vi "Teleop.vi"(10 "Match Info":T1={"Autonomous Elapsed Seconds"=0.0, "TeleOp Elapsed Seconds"=0.0, "Disabled Elapsed Seconds"=0.0, "Visited Autonomous"=FALSE, "Visited TeleOp"=FALSE, "Visited Disabled"=FALSE, "Autonomous Settings"={"Autonomous Style"=enum."Independent", "VI Refnum"=refnum}}, 11 "Call Context":T2) -> ()   [LabVIEW 2017]
doc: "This VI is called for each TeleOp packet received from the DS where the robot is not disabled. It is often used to read from the joysticks and update I/O or to update setpoints for timed control loops. It should complete and return within 20 milliseconds or it may miss DS packets."
uses:
  <vilib>/Rock Robotics/WPI/DriverStation/WPI_DriverStationDerivedRobotMode.ctl
  <vilib>/Rock Robotics/WPI/DriverStation/WPI_DriverStationMatch Info.ctl
  <vilib>/Rock Robotics/WPI/Solenoid/WPI_SolenoidValue.ctl
  <vilib>/Rock Robotics/WPI/ThirdParty/Phoenix-LabVIEW/Motor Controller/Controls/CTRE_Phoenix_MotorControl_ControlMode.ctl
  <vilib>/Rock Robotics/WPI/Utilities/WPI_GetSetVariantRefNum.vi
  <vilib>/Rock Robotics/WPI/Solenoid/WPI_SolenoidSetEnum.vi
  <vilib>/Rock Robotics/Network Tables/NT Write Boolean Array.vi
  <vilib>/Rock Robotics/Network Tables/NT Write Numeric Array.vi
  <vilib>/Rock Robotics/Network Tables/NT Read Boolean.vi
  <vilib>/Rock Robotics/Network Tables/NT Read Number.vi
  Robot Global Data.vi
  <vilib>/addons/control/pid/NI_PID_pid.lvlib
  <vilib>/addons/control/pid/pid.llb/PID (DBL).vi
panel:
  out "Claw Status":bool
  out "AbsArm":dbl
  out "Sample Slider 0":dbl(slide) scale=0.0..5.0
  out "Sample Boolean 1":bool
  out "Sample Boolean 0":bool
  # "TUSKS"
  # "Axis 1"
  # "DRIVE"
  # "Axis 1"
  # "PULSE"
  # "Button 3"
  # "Button 3"
  # "Axis 0"
  # "Axis 0"
  # "Button 2"
  # "Button 1"
  # "Button 2"
  # "Button 1"
  # "Button 0"
  # "Button 0"
  # "CONTROLLER  LAYOUT"
  # "CONTROLLER  LAYOUT"
  # "Joystick 1"
  # "Joystick 0"
  # "Joystick 1"
  # "https://www.xbox.com/en-us/xbox-one/accessories"
  # "Axis 4"
  # "Axis 4"
  # "DRIVE TURN"
  # "Left"
  # "Left"
  # "Axis 5"
  # "Axis 5"
  # "CLAW IN"
  # "Button 4"
  # "ELBOW DOWN"
  # "Button 4"
  # "Axis 2"
  # "ARM DOWN"
  # "Axis 2"
  # "BELT IN"
  # "Right"
  # "Button 5"
  # "ELBOW UP"
  # "Button 5"
  # "CLAW OUT"
  # "Axis 3"
  # "ARM UP"
  # "Axis 3"
  # "BELT OUT"
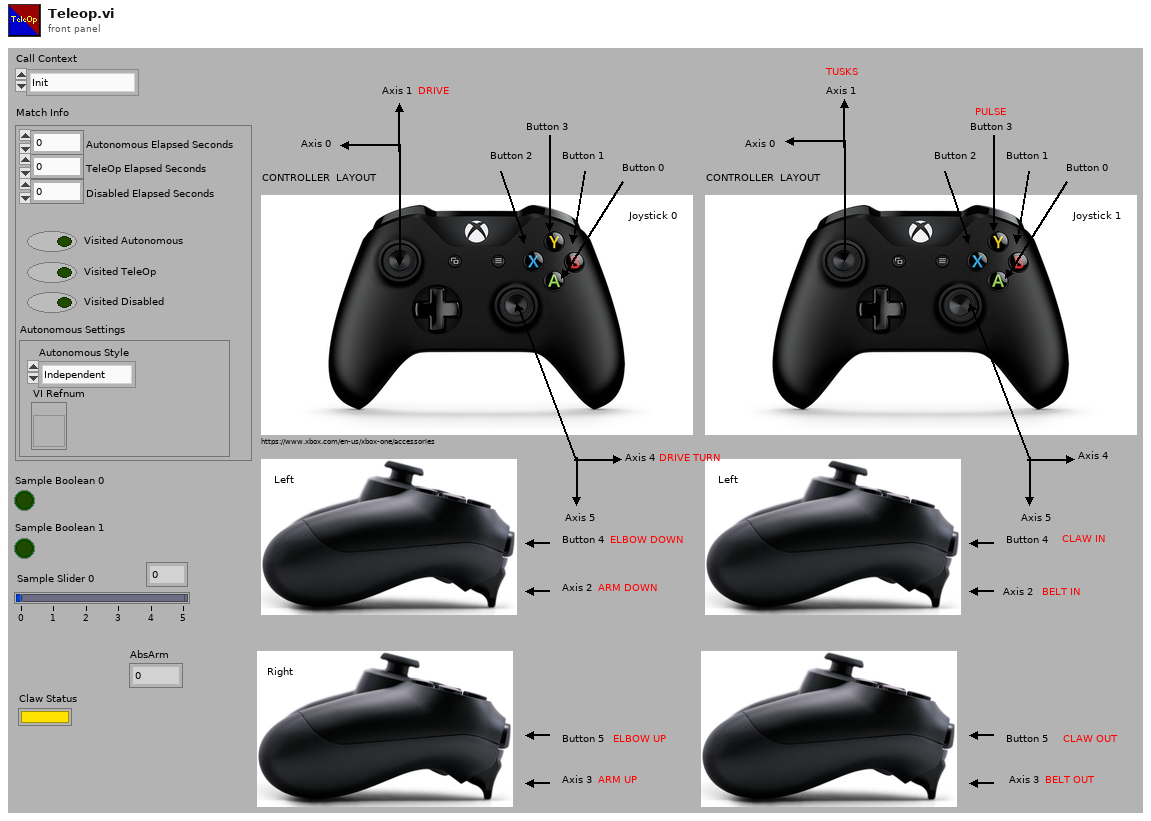
[diagram p1: front panel]
types:
  T1 = typedef "WPI_DriverStationMatch Info.ctl" = cluster{"Autonomous Elapsed Seconds":dbl, "TeleOp Elapsed Seconds":dbl, "Disabled Elapsed Seconds":dbl, "Visited Autonomous":bool, "Visited TeleOp":bool, "Visited Disabled":bool, "Autonomous Settings":cluster{"Autonomous Style":enum16{"Iterative", "Independent"}, "VI Refnum":refnum<vi>}}
  T2 = typedef "WPI_DriverStationDerivedRobotMode.ctl" = enum16{"Init", "Execute", "Stop"}
  T3 = typedef "WPI_JoystickDevRef.ctl" = cluster{"Device":T4}
  T4 = typedef "WPI_JoystickDeviceEnum.ctl" = enum16{"USB 0", "USB 1", "USB 2", "USB 3", "USB 4", "USB 5"}
  T5 = cluster{"Axes[0]":dbl, "Axes[1]":dbl, "Axes[2]":dbl, "Axes[3]":dbl, "Axes[4]":dbl, "Axes[5]":dbl, "Axes[6]":dbl, "Axes[7]":dbl, "Axes[8]":dbl}
  T6 = cluster{"Buttons[0]":bool, "Buttons[1]":bool, "Buttons[2]":bool, "Buttons[3]":bool, "Buttons[4]":bool, "Buttons[5]":bool, "Buttons[6]":bool, "Buttons[7]":bool, "Buttons[8]":bool}
  T7 = typedef "CTRE_Phoenix_MotorControl_ControlMode.ctl" = u16
  T8 = typedef "WPI_MotorControlDeviceRef.ctl" = cluster{"DeviceStatus":errorcluster, "Type":T9, "PWM":cluster{"PWM Channel":T10, "DeadBand":T11}, "CAN":cluster{"Device Number":u8, "SetOutput VI Ref":variant, "GetOutput VI Ref":variant, "Enable VI Ref":variant, "Disable VI Ref":variant, "Data":variant}, "Invert":bool, "DIO PWM":cluster{"PWM \"Enable\" Channel":T10, "DIOChannel":T12, "PWM Rate":dbl}}
  T9 = typedef "WPI_MotorControlType.ctl" = enum16{"PWM", "CAN", "DIO PWM"}
  T10 = typedef "FPGA_DIOPWMChannel.ctl" = enum8{"PWM 0", "PWM 1", "PWM 2", "PWM 3", "PWM 4", "PWM 5", "PWM 6", "PWM 7", "PWM 8", "PWM 9", "PWM MXP 0", "PWM MXP 1", "PWM MXP 2", "PWM MXP 3", "PWM MXP 4", "PWM MXP 5", "PWM MXP 6", "PWM MXP 7", "PWM MXP 8", "PWM MXP 9", "Invalid"}
  T11 = typedef "WPI_PWMDeadband.ctl" = cluster{"Name":string, "maxPositivePwm":i32, "minPositivePwm":i32, "centerPwm":i32, "maxNegativePwm":i32, "minNegativePwm":i32, "angularRange":u16}
  T12 = typedef "FPGA_DIOChannel.ctl" = enum8{"DIO 0", "DIO 1", "DIO 2", "DIO 3", "DIO 4", "DIO 5", "DIO 6", "DIO 7", "DIO 8", "DIO 9", "DIO MXP 0", "DIO MXP 1", "DIO MXP 2", "DIO MXP 3", "DIO MXP 4", "DIO MXP 5", "DIO MXP 6", "DIO MXP 7", "DIO MXP 8", "DIO MXP 9", "DIO MXP 10", "DIO MXP 11", "DIO MXP 12", "DIO MXP 13", "DIO MXP 14", "DIO MXP 15", "SPI Port CS1", "SPI Port CS2", "SPI Port CS3", "SPI Port MISO", "SPI Port MOSI", "Invalid"}
  T13 = typedef "WPI_SolenoidValue.ctl" = enum16{"Off", "On", "Forward", "Reverse"}
  T14 = typedef "WPI_SolenoidDevRef.ctl" = cluster{"DevStatus":errorcluster, "Pneumatics Control Module":u8, "Forward Solenoid Channel":T15, "Reverse Solenoid Channel":T15}
  T15 = typedef "WPI_SolenoidChannel.ctl" = enum8{"Solenoid 0", "Solenoid 1", "Solenoid 2", "Solenoid 3", "Solenoid 4", "Solenoid 5", "Solenoid 6", "Solenoid 7", "Invalid"}
  T16 = enum16{"Arm Down", "Arm Switch", "Arm(Low Scale)", "Arm(Normal Scale)", "Arm(High Scale)", "Hang"}
  T17 = cluster{"proportional gain (Kc)":dbl, "integral time (Ti, min)":dbl, "derivative time (Td, min)":dbl}
  T18 = enum16{"Arm Down", "Arm Switch", "Arm(Low Scale)", "Arm(Normal Scale)", "Arm(High Scale)"}
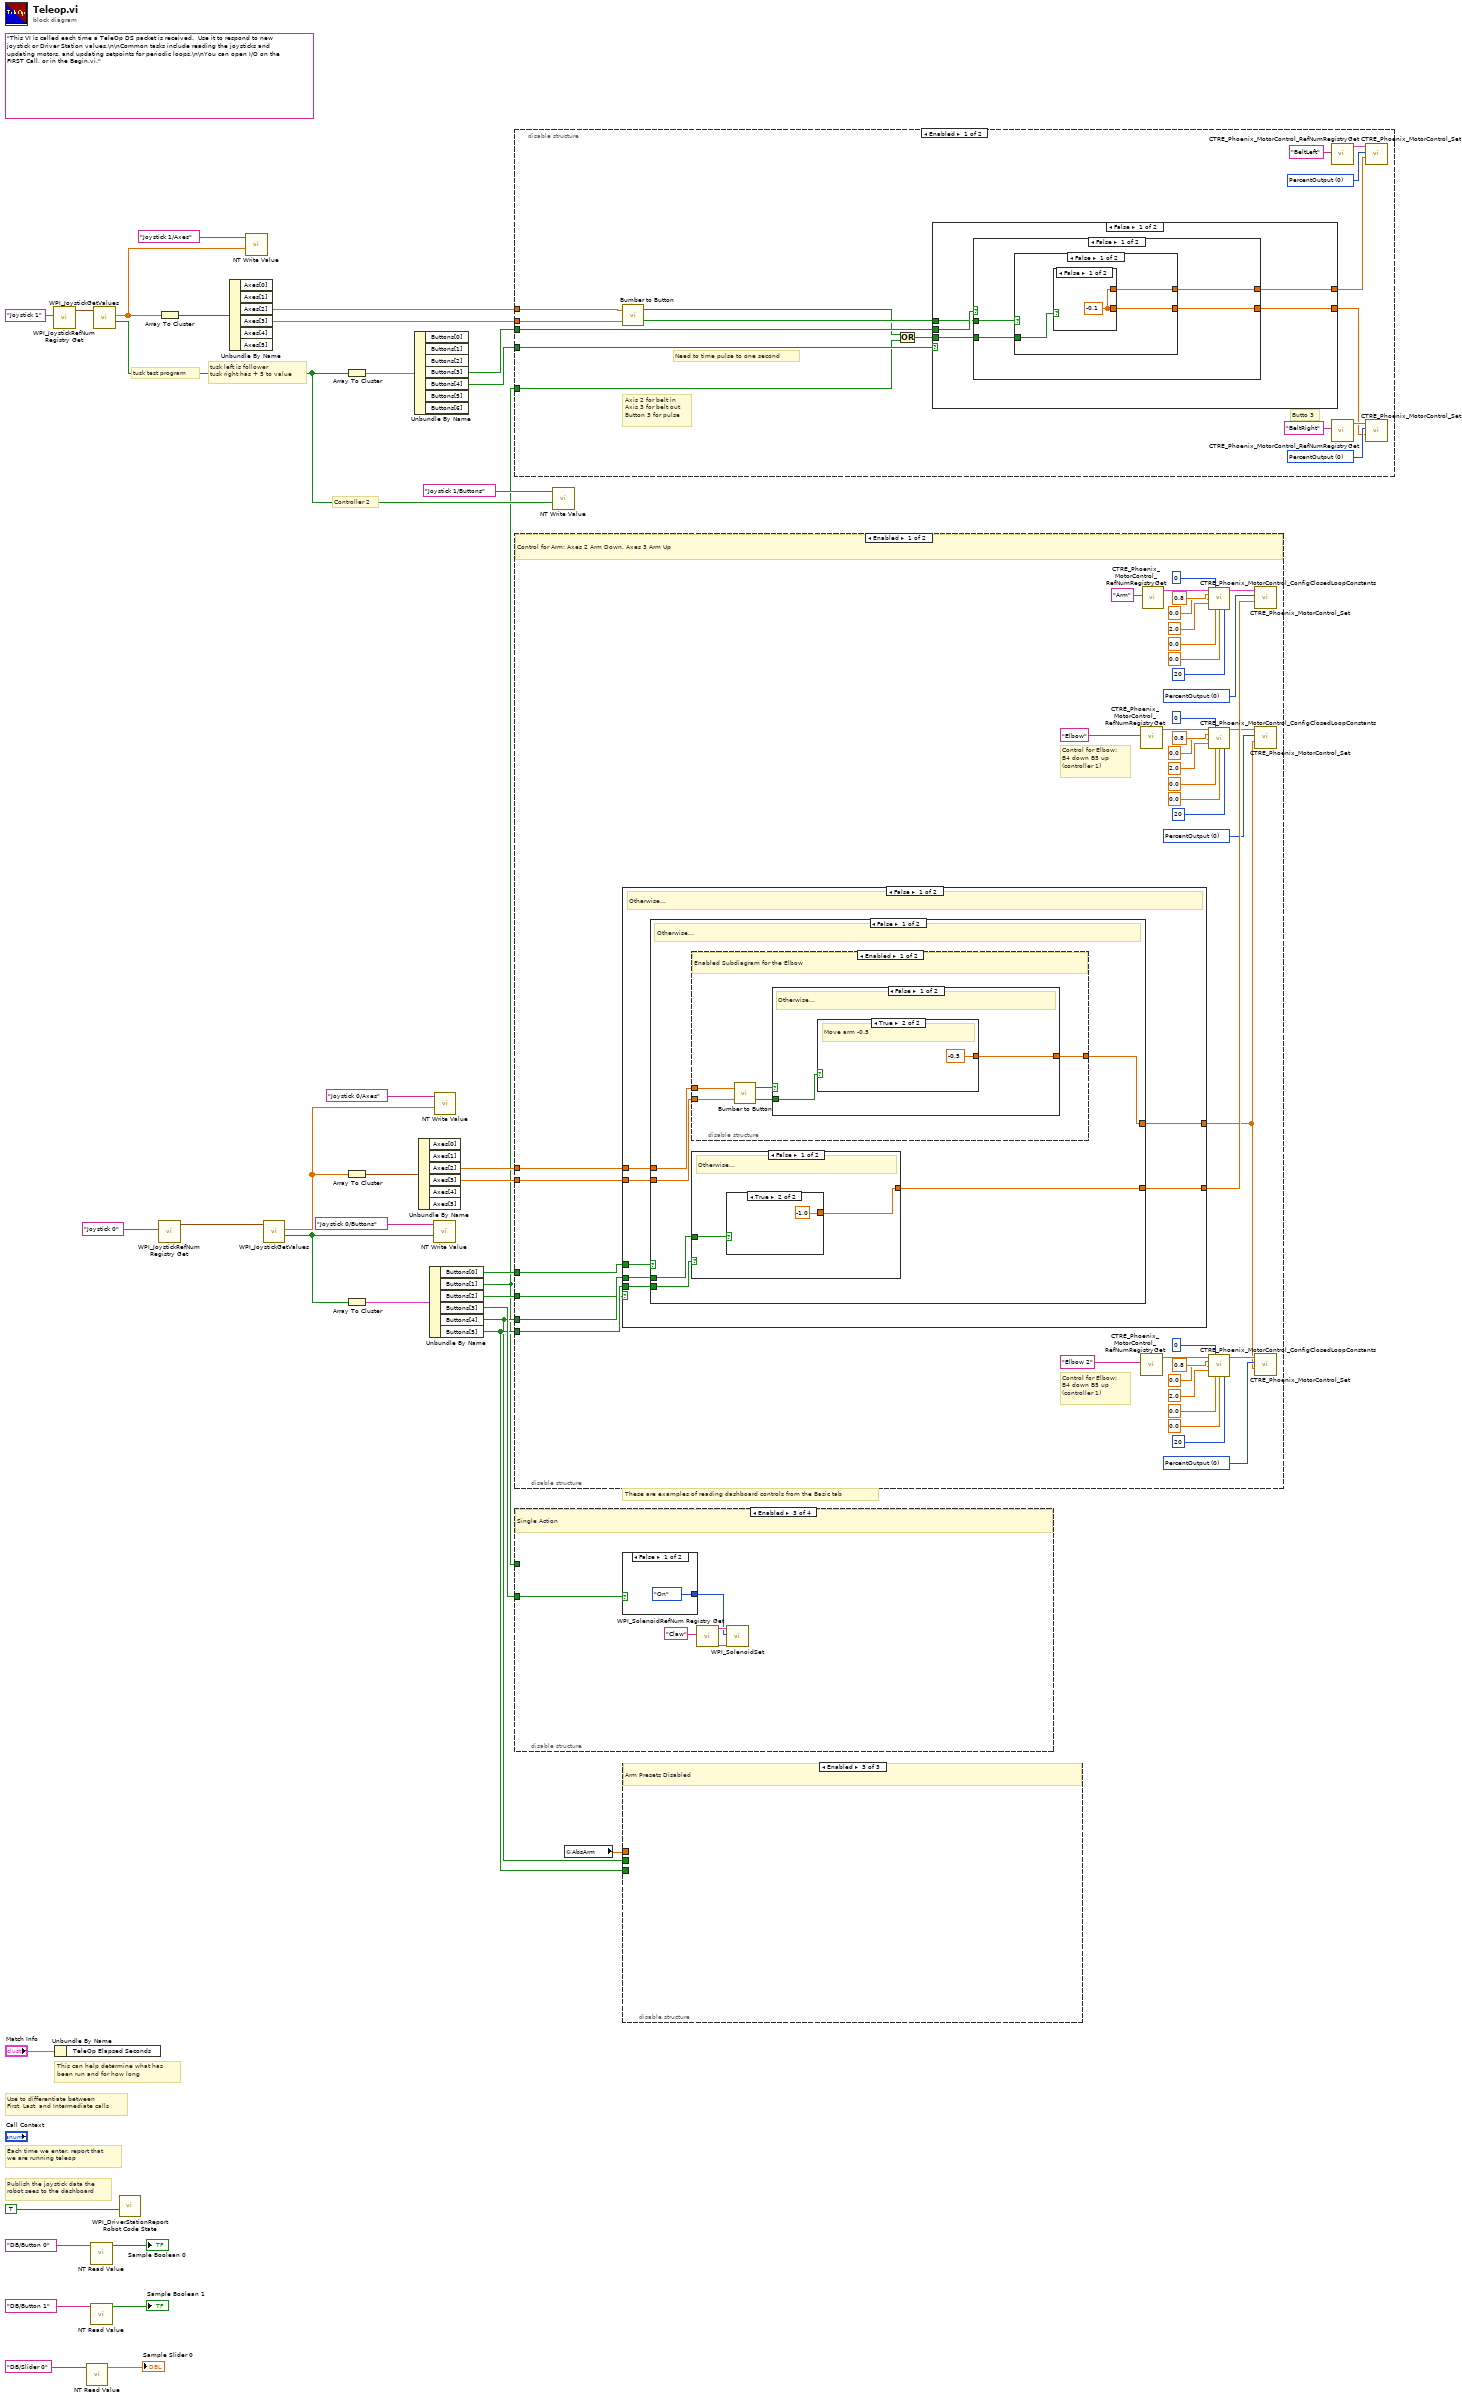
[diagram p0: block diagram]
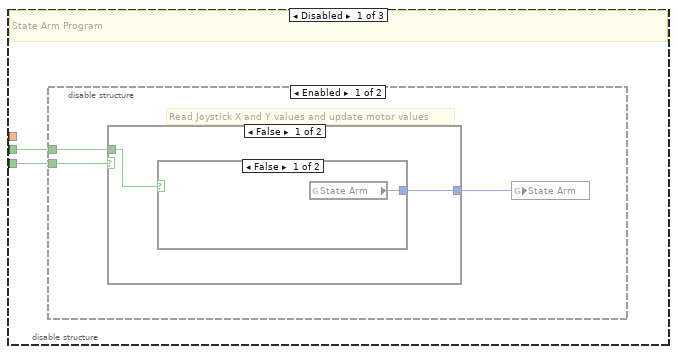
[diagram p2: hidden frame]
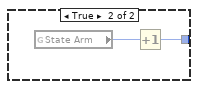
[diagram p3: hidden frame]
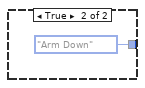
[diagram p4: hidden frame]
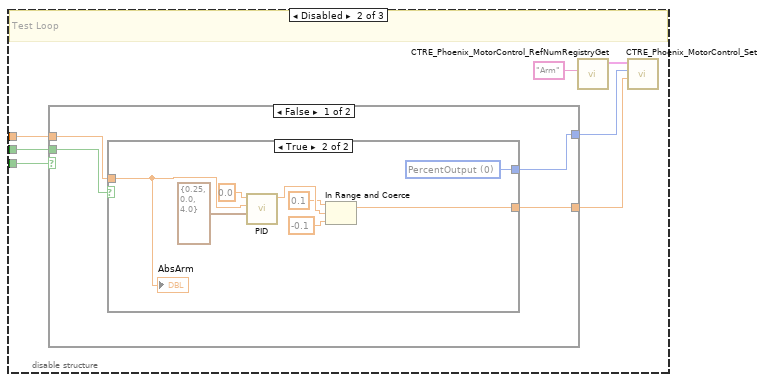
[diagram p6: hidden frame]
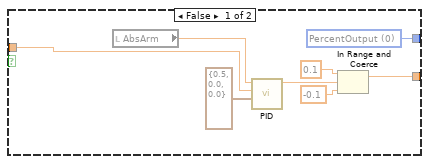
[diagram p7: hidden frame]
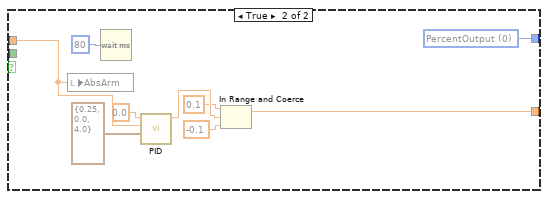
[diagram p8: hidden frame]
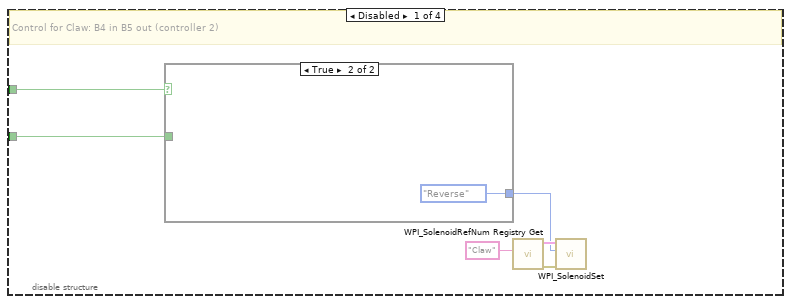
[diagram p9: hidden frame]
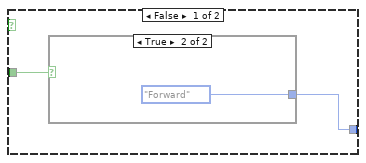
[diagram p10: hidden frame]
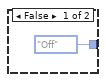
[diagram p11: hidden frame]
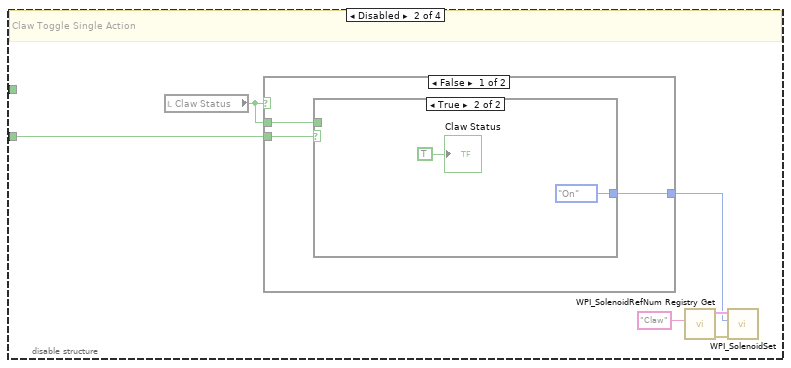
[diagram p12: hidden frame]
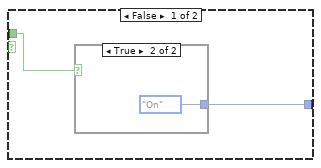
[diagram p13: hidden frame]
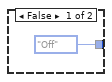
[diagram p14: hidden frame]
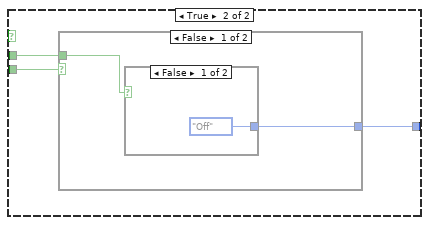
[diagram p15: hidden frame]
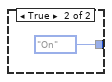
[diagram p16: hidden frame]
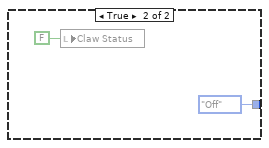
[diagram p17: hidden frame]
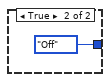
[diagram p18: hidden frame]
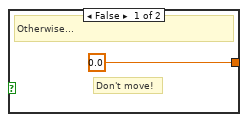
[diagram p20: hidden frame]
diagram:
  (unwired) "This VI is called each time a TeleOp DS packet is received.  Use it to respond to new joystick or Driver Station values.\n\nCommon tasks include reading the joysticks and updating motors, and updating setpoints for periodic loops.\n\nYou can open I/O on the FIRST Call, or in the Begin.vi."
  # "tusk left is follower\ntusk right has + 5 to value"
  # "tusk test program"
  # "Controller 2"
  # "These are examples of reading dashboard controls from the Basic tab"
  # "Publish the joystick data the\nrobot sees to the dashboard"
  # "Each time we enter, report that\nwe are running teleop"
  # "Use to differentiate between\nFirst, Last, and Intermediate calls"
  # "This can help determine what has\nbeen run and for how long"
  n1 = call <vilib>:"WPI_JoystickRefNum Registry Get.vi"("refnum name"="Joystick 1") -> ("JoystickDevRef"=w21:T3)  [unwired: 9 in, 1 out]
  n2 = Unbundle By Name("Match Info") -> ()  [unwired: 1 out]
  n3 = call-poly <vilib>:"NT Read Value.vi"("Name"="DB/Slider 0" ("refnum name")) -> ("Numeric"=→"Sample Slider 0":dbl)  [unwired: 9 in, 1 out]
  n4 = call-poly <vilib>:"NT Read Value.vi"("Name"="DB/Button 0" ("refnum name")) -> ("Boolean"=→"Sample Boolean 0":bool)  [unwired: 9 in, 1 out]
  n5 = call-poly <vilib>:"NT Read Value.vi"("Name"="DB/Button 1" ("refnum name")) -> ("Boolean"=→"Sample Boolean 1":bool)  [unwired: 9 in, 1 out]
  n6 = call <vilib>:"WPI_JoystickGetValues.vi"("JoystickDevRef"=w21) -> ("Buttons"=w16:bool[], "Axes"=w15:dbl[])  [unwired: 6 in, 3 out]
  n7 = call <vilib>:"WPI_DriverStationReport Robot Code State.vi"("TeleOp"=TRUE ("Autonomous")) -> ()  [unwired: 10 in, 1 out]
  n8 = Array To Cluster(array=w15) -> (cluster=w19:T5)
  n9 = call <vilib>:"WPI_JoystickRefNum Registry Get.vi"("refnum name"="Joystick 0") -> ("JoystickDevRef"=w35:T3)  [unwired: 1 in, 9 out]
  n10 = Unbundle By Name(w19) -> ("Axes[2]"=w11:dbl, "Axes[3]"=w12:dbl)  [unwired: 4 out]
  n11 = call-poly <vilib>:"NT Write Value.vi"("Numeric Array"=w15, "Name"="Joystick 1/Axes") -> ()  [unwired: 9 in, 1 out]
  n12 = call <vilib>:"WPI_JoystickGetValues.vi"("JoystickDevRef"=w35) -> ("Buttons"=w23:bool[], "Axes"=w25:dbl[])  [unwired: 6 in, 3 out]
  n13 = Array To Cluster(array=w16) -> (cluster=w18:T6)
  n14 = Array To Cluster(array=w25) -> (cluster=w24:T5)
  n15 = Array To Cluster(array=w23) -> (cluster=w22:T6)
  n16 = Unbundle By Name(w18) -> ("Buttons[3]"=w13:bool, "Buttons[4]"=w2:bool)  [unwired: 5 out]
  n17 = Unbundle By Name(w24) -> ("Axes[2]"=w5:dbl, "Axes[3]"=w4:dbl)  [unwired: 4 out]
  n18 = Unbundle By Name(w22) -> ("Buttons[0]"=w3:bool, "Buttons[1]"=w1:bool, "Buttons[2]"=w8:bool, "Buttons[3]"=w9:bool, "Buttons[4]"=w6:bool, "Buttons[5]"=w7:bool)
  n19 = call-poly <vilib>:"NT Write Value.vi"("Boolean Array"=w23, "Name"="Joystick 0/Buttons") -> ()  [unwired: 9 in, 1 out]
  n20 = call-poly <vilib>:"NT Write Value.vi"("Numeric Array"=w25, "Name"="Joystick 0/Axes") -> ()  [unwired: 9 in, 1 out]
  n21 = disable-structure shown="Enabled" {
    disable-tunnel: w13 -> [w46 _]
    disable-tunnel: w12 -> [w45 _]
    disable-tunnel: w11 -> [w44 _]
    disable-tunnel: w2 -> [w42 _]
    disable-tunnel: w1 -> [w38 _]
    frame Enabled {
      w48 = T7 0 items=["PercentOutput"=0, "Position"=1, "Velocity"=2, "Current"=3, "Follower"=5, "MotionProfile"=6, "MotionMagic"=7, "MotionMagicArc"=8, "MotionProfileArc"=10, "Disabled"=15] ("Control Mode")
      w49 = T7 0 items=["PercentOutput"=0, "Position"=1, "Velocity"=2, "Current"=3, "Follower"=5, "MotionProfile"=6, "MotionMagic"=7, "MotionMagicArc"=8, "MotionProfileArc"=10, "Disabled"=15] ("Control Mode")
      # "Axis 2 for belt in\nAxis 3 for belt out\nButton 3 for pulse"
      # "Butto 3"
      # "Need to time pulse to one second"
      n22 = call "Bumber to Button.vi"("Bumper / Axis 2"=w45, "Bumper / Axis 1"=w44) -> ("Boolean Output 2"=w43:bool, "Boolean Output 1"=w39:bool)
      n23 = Or(x=w39, y=w38) -> (x .or. y?=w40:bool)
      n24 = case shown="False" w42 {
        tunnel: [w58 w71] -> w41
        tunnel: [w57 w71] -> w47
        tunnel: w46 -> [w56 _]
        tunnel: w43 -> [w55 _]
        tunnel: w40 -> [w54 _]
        frame False {
          n25 = case shown="False" w56 {
            tunnel: [w62 1.0 ("Output")] -> w57
            tunnel: [w61 -1.0 ("Output")] -> w58
            tunnel: w55 -> [w60 _]
            tunnel: w54 -> [w59 _]
            frame False {
              n26 = case shown="False" w60 {
                tunnel: [w65 w68] -> w62
                tunnel: [w64 w68] -> w61
                tunnel: w59 -> [w63 _]
                frame False {
                  n27 = case shown="False" w63 {
                    tunnel: [w66 w67] -> w65
                    tunnel: [w66 w67] -> w64
                    frame False {
                      w66 = -0.1 ("Output")
                    }
                    frame True {
                      w67 = 1.0 ("Output")
                    }
                  }
                }
                frame True {
                  w68 = -1.0 ("Output")
                }
              }
            }
            frame True {
            }
          }
        }
        frame True {
          w71 = 1.0 ("Output")
        }
      }
      n28 = call <vilib>:"CTRE_Phoenix_MotorControl_RefNumRegistryGet.vi"("refnum name"="BeltLeft") -> ("PhoenixMotorControlDevRef"=w53:T8)  [unwired: 9 in, 1 out]
      n29 = call <vilib>:"CTRE_Phoenix_MotorControl_RefNumRegistryGet.vi"("refnum name"="BeltRight") -> ("PhoenixMotorControlDevRef"=w52:T8)  [unwired: 9 in, 1 out]
      n30 = call <vilib>:"CTRE_Phoenix_MotorControl_Set.vi"("Output"=w47, "Control Mode"=w48, "PhoenixMotorControlDevRef"=w53) -> ()  [unwired: 7 in, 2 out]
      n31 = call <vilib>:"CTRE_Phoenix_MotorControl_Set.vi"("Output"=w41, "Control Mode"=w49, "PhoenixMotorControlDevRef"=w52) -> ()  [unwired: 7 in, 2 out]
    }
    frame Disabled {
    }
  }
  n32 = disable-structure "Diagram Disable Structure" shown="Enabled" {
    disable-tunnel: w8 -> [w84 _]
    disable-tunnel: w7 -> [w101 _]
    disable-tunnel: w6 -> [w100 _]
    disable-tunnel: w5 -> [w97 _]
    disable-tunnel: w4 -> [w98 _]
    disable-tunnel: w3 -> [w85 _]
    frame Enabled {
      w74 = T7 0 items=["PercentOutput"=0, "Position"=1, "Velocity"=2, "Current"=3, "Follower"=5, "MotionProfile"=6, "MotionMagic"=7, "MotionMagicArc"=8, "MotionProfileArc"=10, "Disabled"=15] ("Control Mode")
      w87 = T7 0 items=["PercentOutput"=0, "Position"=1, "Velocity"=2, "Current"=3, "Follower"=5, "MotionProfile"=6, "MotionMagic"=7, "MotionMagicArc"=8, "MotionProfileArc"=10, "Disabled"=15] ("Control Mode")
      w111 = T7 0 items=["PercentOutput"=0, "Position"=1, "Velocity"=2, "Current"=3, "Follower"=5, "MotionProfile"=6, "MotionMagic"=7, "MotionMagicArc"=8, "MotionProfileArc"=10, "Disabled"=15] ("Control Mode")
      # "Control for Elbow:\nB4 down B5 up\n(controller 1)"
      # "Control for Elbow:\nB4 down B5 up\n(controller 1)"
      # "Control for Arm: Axes 2 Arm Down, Axes 3 Arm Up"
      n33 = case shown="False" w84 {
        tunnel: w85 -> [w119 _]
        tunnel: w101 -> [w118 _]
        tunnel: w100 -> [w117 _]
        tunnel: [w116 0.7 ("Output")] -> w99
        tunnel: w98 -> [w115 _]
        tunnel: w97 -> [w114 _]
        tunnel: [w113 -1.0 ("Output")] -> w72
        frame False {
          # "Otherwise..."
          n34 = case shown="False" w119 {
            tunnel: w118 -> [w125 _]
            tunnel: w117 -> [w124 _]
            tunnel: [w123 -0.7 ("Output")] -> w116
            tunnel: w115 -> [w121 _]
            tunnel: w114 -> [w122 _]
            tunnel: [w120 1.0 ("Output")] -> w113
            frame False {
              # "Otherwise..."
              n35 = disable-structure "Diagram Disable Structure" shown="Enabled" {
                disable-tunnel: w122 -> [w128 _]
                disable-tunnel: w121 -> [w127 _]
                disable-tunnel: [w126 _] -> w120
                frame Enabled {
                  # "Enabled Subdiagram for the Elbow"
                  n36 = call "Bumber to Button.vi"("Bumper / Axis 2"=w127, "Bumper / Axis 1"=w128) -> ("Boolean Output 2"=w129:bool, "Boolean Output 1"=w130:bool)
                  n37 = case shown="False" w130 {
                    tunnel: [w132 1.0 ("Output")] -> w126
                    tunnel: w129 -> [w131 _]
                    frame False {
                      # "Otherwise..."
                      n38 = case shown="True" w131 {
                        tunnel: [0.0 ("Output") -0.5 ("Output")] -> w132
                        frame False {
                          # "Don't move!"
                          # "Otherwise..."
                        }
                        frame True {
                          # "Move arm -0.5"
                        }
                      }
                    }
                    frame True {
                      # "Move elbow UP"
                    }
                  }
                }
                frame Disabled {
                  # "Disabled Elbow diagram"
                }
              }
              n39 = case shown="False" w125 {
                tunnel: [w137 1.0 ("Output")] -> w123
                tunnel: w124 -> [w136 _]
                frame False {
                  # "Otherwise..."
                  n40 = case shown="True" w136 {
                    tunnel: [0.0 ("Output") -1.0 ("Output")] -> w137
                    frame False {
                    }
                    frame True {
                    }
                  }
                }
                frame True {
                  # "Move arm UP"
                }
              }
            }
            frame True {
              # "Move arm 1 and elbow -0.6  (same speed)"
            }
          }
        }
        frame True {
          # "If true, arm -1, elbow 0.6 (same speed)"
        }
      }
      n41 = call <vilib>:"CTRE_Phoenix_MotorControl_RefNumRegistryGet.vi"("refnum name"="Elbow") -> ("PhoenixMotorControlDevRef"=w95:T8)  [unwired: 9 in, 1 out]
      n42 = call <vilib>:"CTRE_Phoenix_MotorControl_RefNumRegistryGet.vi"("refnum name"="Elbow 2") -> ("PhoenixMotorControlDevRef"=w82:T8)  [unwired: 9 in, 1 out]
      n43 = call <vilib>:"CTRE_Phoenix_MotorControl_RefNumRegistryGet.vi"("refnum name"="Arm") -> ("PhoenixMotorControlDevRef"=w110:T8)  [unwired: 9 in, 1 out]
      n44 = call <vilib>:"CTRE_Phoenix_MotorControl_ConfigClosedLoopConstants.vi"("PhoenixMotorControlDevRef"=w110, "slotIdx"=0, "P"=0.8, "I"=0.0, "D"=2.0, "F"=0.0, "I Zone"=0.0, "timeoutMs"=20) -> ("PhoenixMotorControlDevRef"=w109:T8)  [unwired: 6 in, 1 out]
      n45 = call <vilib>:"CTRE_Phoenix_MotorControl_ConfigClosedLoopConstants.vi"("PhoenixMotorControlDevRef"=w95, "slotIdx"=0, "P"=0.8, "I"=0.0, "D"=2.0, "F"=0.0, "I Zone"=0.0, "timeoutMs"=20) -> ("PhoenixMotorControlDevRef"=w96:T8)  [unwired: 6 in, 1 out]
      n46 = call <vilib>:"CTRE_Phoenix_MotorControl_ConfigClosedLoopConstants.vi"("PhoenixMotorControlDevRef"=w82, "slotIdx"=0, "P"=0.8, "I"=0.0, "D"=2.0, "F"=0.0, "I Zone"=0.0, "timeoutMs"=20) -> ("PhoenixMotorControlDevRef"=w83:T8)  [unwired: 6 in, 1 out]
      n47 = call <vilib>:"CTRE_Phoenix_MotorControl_Set.vi"("Output"=w99, "Control Mode"=w111, "PhoenixMotorControlDevRef"=w109) -> ()  [unwired: 7 in, 2 out]
      n48 = call <vilib>:"CTRE_Phoenix_MotorControl_Set.vi"("Output"=w72, "Control Mode"=w87, "PhoenixMotorControlDevRef"=w96) -> ()  [unwired: 7 in, 2 out]
      n49 = call <vilib>:"CTRE_Phoenix_MotorControl_Set.vi"("Output"=w72, "Control Mode"=w74, "PhoenixMotorControlDevRef"=w83) -> ()  [unwired: 7 in, 2 out]
    }
    frame Disabled {
      # "Arm Disabled"
    }
  }
  n50 = disable-structure "Diagram Disable Structure" shown="Enabled" {
    disable-tunnel: w9 -> [w147 w158 w180 _]
    disable-tunnel: w1 -> [w145 _ _ _]
    frame Disabled {
      # "Control for Claw: B4 in B5 out (controller 2)"
      n51 = case shown="True" w145 {
        tunnel: w147 -> [w152 _]
        tunnel: [w151 WPI_SolenoidValue."Reverse" ("Value")] -> w146
        frame False {
          n52 = case shown="True" w152 {
            tunnel: [WPI_SolenoidValue."Off" ("Value") WPI_SolenoidValue."Forward" ("Value")] -> w151
            frame False {
            }
            frame True {
            }
          }
        }
        frame True {
        }
      }
      n53 = call <vilib>:"WPI_SolenoidRefNum Registry Get.vi"("refnum name"="Claw") -> ("error out"=w149:errorcluster, "SolenoidDevRef"=w150:T14)  [unwired: 9 in]
      n54 = call-poly <vilib>:"WPI_SolenoidSet.vi"("error in (no error)"=w149, "Value"=w146, "SolenoidDevRef"=w150) -> ()  [unwired: 7 in, 2 out]
    }
    frame Disabled {
      # "Claw Toggle Single Action"
      n55 = local read "Claw Status"() -> (w157:bool)
      n56 = case shown="False" w157 {
        tunnel: w158 -> [w164 w173]
        tunnel: w157 -> [w163 w172]
        tunnel: [w162 w171] -> w156
        frame False {
          n57 = case shown="True" w164 {
            tunnel: w163 -> [w166 _]
            tunnel: [w165 WPI_SolenoidValue."On" ("Value")] -> w162
            frame False {
              n58 = case shown="True" w166 {
                tunnel: [WPI_SolenoidValue."Off" ("Value") WPI_SolenoidValue."On" ("Value")] -> w165
                frame False {
                }
                frame True {
                }
              }
            }
            frame True {
              "Claw Status" <- TRUE
            }
          }
        }
        frame True {
          n59 = case shown="False" w173 {
            tunnel: w172 -> [w175 _]
            tunnel: [w174 WPI_SolenoidValue."Off" ("Value")] -> w171
            frame False {
              n60 = case shown="False" w175 {
                tunnel: [WPI_SolenoidValue."Off" ("Value") WPI_SolenoidValue."On" ("Value")] -> w174
                frame False {
                }
                frame True {
                }
              }
            }
            frame True {
              n61 = local write "Claw Status"(FALSE ("Boolean")) -> ()
            }
          }
        }
      }
      n62 = call <vilib>:"WPI_SolenoidRefNum Registry Get.vi"("refnum name"="Claw") -> ("error out"=w160:errorcluster, "SolenoidDevRef"=w161:T14)  [unwired: 9 in]
      n63 = call-poly <vilib>:"WPI_SolenoidSet.vi"("error in (no error)"=w160, "Value"=w156, "SolenoidDevRef"=w161) -> ()  [unwired: 7 in, 2 out]
    }
    frame Enabled {
      # "Single Action"
      n64 = case shown="False" w180 {
        tunnel: [WPI_SolenoidValue."On" ("Value") WPI_SolenoidValue."Off" ("Value")] -> w181
        frame False {
        }
        frame True {
        }
      }
      n65 = call <vilib>:"WPI_SolenoidRefNum Registry Get.vi"("refnum name"="Claw") -> ("error out"=w183:errorcluster, "SolenoidDevRef"=w184:T14)  [unwired: 9 in]
      n66 = call-poly <vilib>:"WPI_SolenoidSet.vi"("error in (no error)"=w183, "Value"=w181, "SolenoidDevRef"=w184) -> ()  [unwired: 7 in, 2 out]
    }
    frame Disabled {
      # "Claw Disabled"
    }
  }
  n67 = call-poly <vilib>:"NT Write Value.vi"("Boolean Array"=w16, "Name"="Joystick 1/Buttons") -> ()  [unwired: 9 in, 1 out]
  n68 = global read "Robot Global Data.vi" "AbsArm"() -> (w10:dbl)
  n69 = disable-structure shown="Enabled" {
    disable-tunnel: w10 -> [_ w202 _]
    disable-tunnel: w6 -> [w187 w199 _]
    disable-tunnel: w7 -> [w188 w198 _]
    frame Disabled {
      # "State Arm Program"
      n70 = disable-structure shown="Enabled" {
        disable-tunnel: w188 -> [w190 _]
        disable-tunnel: w187 -> [w189 _]
        frame Enabled {
          # "Read Joystick X and Y values and update motor values"
          n71 = case shown="False" w190 {
            tunnel: [w193 T16."Arm Down" ("State Arm")] -> w191
            tunnel: w189 -> [w192 _]
            frame False {
              n72 = case shown="False" w192 {
                tunnel: [w194 w195] -> w193
                frame False {
                  n73 = global read "Robot Global Data.vi" "State Arm"() -> (w194:T18)
                }
                frame True {
                  n74 = global read "Robot Global Data.vi" "State Arm"() -> (w196:T18)
                  n75 = Increment(x=w196) -> (x+1=w195:T18)
                }
              }
            }
            frame True {
            }
          }
          n76 = global write "Robot Global Data.vi" "State Arm"(w191) -> ()
        }
        frame Disabled {
        }
      }
    }
    frame Disabled {
      # "Test Loop"
      n77 = case shown="False" w198 {
        tunnel: [w208 w227] -> w200
        tunnel: [w206 w226] -> w201
        tunnel: w202 -> [w207 w225]
        tunnel: w199 -> [w205 _]
        frame False {
          n78 = case shown="True" w205 {
            tunnel: [w216 w220] -> w206
            tunnel: [w213 w219] -> w208
            tunnel: w207 -> [w210 w217]
            frame False {
              w216 = T7 0 items=["PercentOutput"=0, "Position"=1, "Velocity"=2, "Current"=3, "Follower"=5, "MotionProfile"=6, "MotionMagic"=7, "MotionMagicArc"=8, "MotionProfileArc"=10, "Disabled"=15] ("Control Mode")
              n79 = local read "AbsArm"() -> (w209:dbl)
              n80 = call-poly <vilib>:"PID.vi"("PID gains"=T17 {"proportional gain (Kc)"=0.5, "integral time (Ti, min)"=0.0, "derivative time (Td, min)"=0.0}, "process variable"=w210, "setpoint"=w209) -> ("output"=w211:dbl)  [unwired: 7 in, 1 out]
              n81 = In Range and Coerce(upper limit=0.1, x=w211, lower limit=-0.1) -> (coerced(x)=w213:dbl)  [unwired: 1 out]
            }
            frame True {
              w220 = T7 0 items=["PercentOutput"=0, "Position"=1, "Velocity"=2, "Current"=3, "Follower"=5, "MotionProfile"=6, "MotionMagic"=7, "MotionMagicArc"=8, "MotionProfileArc"=10, "Disabled"=15] ("Control Mode")
              n82 = call-poly <vilib>:"PID.vi"("PID gains"=T17 {"proportional gain (Kc)"=0.25, "integral time (Ti, min)"=0.0, "derivative time (Td, min)"=4.0}, "process variable"=w217, "setpoint"=0.0) -> ("output"=w224:dbl)  [unwired: 7 in, 1 out]
              n83 = In Range and Coerce(upper limit=0.1, x=w224, lower limit=-0.1) -> (coerced(x)=w219:dbl)  [unwired: 1 out]
              "AbsArm" <- w217
            }
          }
        }
        frame True {
          w226 = T7 0 items=["PercentOutput"=0, "Position"=1, "Velocity"=2, "Current"=3, "Follower"=5, "MotionProfile"=6, "MotionMagic"=7, "MotionMagicArc"=8, "MotionProfileArc"=10, "Disabled"=15] ("Control Mode")
          n84 = local write "AbsArm"(w225) -> ()
          n85 = Wait (ms)(milliseconds to wait=u32 80) -> ()  [unwired: 1 out]
          n86 = call-poly <vilib>:"PID.vi"("PID gains"=T17 {"proportional gain (Kc)"=0.25, "integral time (Ti, min)"=0.0, "derivative time (Td, min)"=4.0}, "process variable"=w225, "setpoint"=0.0) -> ("output"=w230:dbl)  [unwired: 7 in, 1 out]
          n87 = In Range and Coerce(upper limit=0.1, x=w230, lower limit=-0.1) -> (coerced(x)=w227:dbl)  [unwired: 1 out]
        }
      }
      n88 = call <vilib>:"CTRE_Phoenix_MotorControl_RefNumRegistryGet.vi"("refnum name"="Arm") -> ("PhoenixMotorControlDevRef"=w203:T8)  [unwired: 9 in, 1 out]
      n89 = call <vilib>:"CTRE_Phoenix_MotorControl_Set.vi"("Output"=w200, "Control Mode"=w201, "PhoenixMotorControlDevRef"=w203) -> ()  [unwired: 7 in, 2 out]
    }
    frame Enabled {
      # "Arm Presets Disabled"
    }
  }
